vi "Change Label Popup.vi"(8 "error in":errorcluster, 11 "Label In":string) -> (0 "error out":errorcluster, 3 "Label Out":string)   [LabVIEW 2019]
doc: "All Rights Reserved © 2017 SyncSols"
uses:
  <vilib>/Utility/inputDevices.llb/keyboardAcquire.vi
panel:
  in  "Label Name":string
  # "<<Enter to Save the Changes>>"
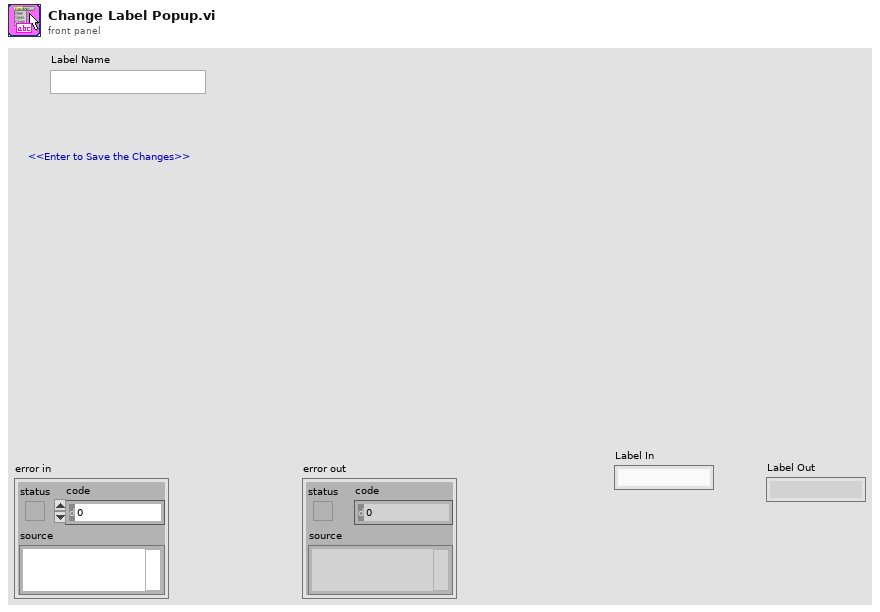
[diagram p1: front panel]
types:
  T1 = enum16{"0", "1", "2", "3", "4", "5", "6", "7", "8", "9", "A", "B", "C", "D", "E", "F", "G", "H", "I", "J", "K", "L", "M", "N", "O", "P", "Q", "R", "S", "T", "U", "V", "W", "X", "Y", "Z", "F1", "F2", "F3", "F4", "F5", "F6", "F7", "F8", "F9", "F10", "F11", "F12", "F13", "F14", "F15", "ADD", "BACK", "BACKSLASH", "CAPITAL", "COMMA", "DECIMAL", "DELETE", "DIVIDE", "DOWN", "END", "EQUALS", "ESCAPE", "GRAVE (`)", "HOME", "INSERT", "LBRACKET", "LCONTROL", "LEFT", "L ALT", "LSHIFT", "LWIN", "MINUS", "MULTIPLY", "NEXT", "NUMLOCK", "NUMPAD_0", "NUMPAD_1", "NUMPAD_2", "NUMPAD_3", "NUMPAD_4", "NUMPAD_5", "NUMPAD_6", "NUMPAD_7", "NUMPAD_8", "NUMPAD_9", "PAUSE", "PERIOD", "PRIOR (PG UP)", "RBRACKET", "RCONTROL", "RETURN", "RIGHT", "R ALT", "RSHIFT", "RWIN", "SCROLL", "SEMICOLON", "SLASH", "SPACE", "SUBTRACT", "TAB", "UP", "ENTER (num pad)", "' (quote)"}
  T2 = enum16{"0", "1", "2", "3", "4", "5", "6", "7", "8", "9", "A", "B", "C", "D", "E", "F", "G", "H", "I", "J", "K", "L", "M", "N", "O", "P", "Q", "R", "S", "T", "U", "V", "W", "X", "Y", "Z", "F1", "F2", "F3", "F4", "F5", "F6", "F7", "F8", "F9", "F10", "F11", "F12", "F13", "F14", "F15", "ADD", "BACK", "BACKSLASH", "CAPITAL", "COMMA", "DECIMAL", "DELETE", "DIVIDE", "DOWN", "END", "EQUALS", "ESCAPE", "GRAVE (`)", "HOME", "INSERT", "LBRACKET", "LCONTROL", "LEFT", "L ALT", "LSHIFT", "LWIN", "MINUS", "MULTIPLY", "NEXT", "NUMLOCK", "NUMPAD_0", "NUMPAD_1", "NUMPAD_2", "NUMPAD_3", "NUMPAD_4", "NUMPAD_5", "NUMPAD_6", "NUMPAD_7", "NUMPAD_8", "NUMPAD_9", "PAUSE", "PERIOD", "PRIOR (PG UP)", "RBRACKET", "RCONTROL", "RETURN", "RIGHT", "R ALT", "RSHIFT", "RWIN", "SCROLL", "SEMICOLON", "SLASH", "SPACE", "SUBTRACT", "TAB", "UP", "ENTER (num pad)", "' (quote)"}[]
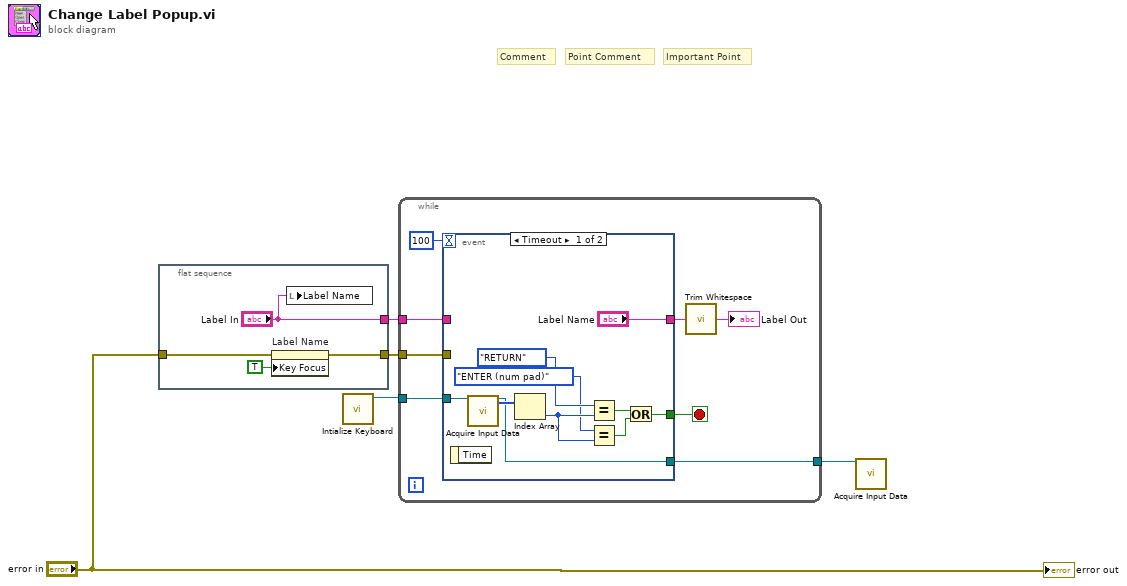
[diagram p0: block diagram]
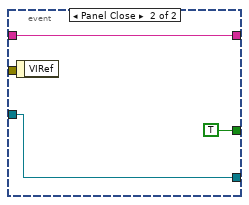
[diagram p2: hidden frame]
diagram:
  # "Important Point"
  # "Point Comment"
  # "Comment"
  n1 = flat-sequence {
    tunnel: "error in" -> [w8]
    tunnel: ["Label In"] -> w4
    tunnel: [w6] -> w1
    frame #0 {
      n2 = property on="Label Name" class="Str"(error in=w8, "Key Focus"=TRUE) -> (error out=w6:errorcluster)  [unwired: 1 in, 1 out]
      n3 = local write "Label Name"("Label In") -> ()
    }
  }
  n4 = call <vilib>:"Intialize Keyboard.vi"() -> ("device ID"=w3:refnum<k1>)  [unwired: 10 in, 1 out]
  n5 = while {
    tunnel: w4 -> [w14]
    tunnel: w3 -> [w13]
    tunnel: [w12] -> w2
    tunnel: w1 -> [w11]
    stop <- w15 stop-if-true
    n6 = event shown="[0] Timeout" {
      selector: _ -> [_ _]
      dyn-events: _ -> [_ _]
      timeout: 100 -> [_ _]
      tunnel: ["Label Name" w29] -> w17
      tunnel: [w21 TRUE] -> w15
      tunnel: w14 -> [_ w29]
      tunnel: w13 -> [w26 w28]
      tunnel: [w18 w28] -> w12
      tunnel: w11 -> [_ _]
      event Timeout {
        n7 = event-data() -> ()  [unwired: 1 in, 1 out]
        n8 = call-poly <vilib>:"Acquire Input Data.vi"("device ID"=w26) -> ("device ID"=w18:refnum<k1>, "keys pressed"=w25:T2)  [unwired: 16 in, 1 out]
        n9 = Index Array(array=w25) -> (element=w23:T1)  [unwired: 1 in]
        n10 = Equal?(x=T1."RETURN" ("keyType 3"), y=w23) -> (x = y?=w20:bool)
        n11 = Equal?(x=T1."ENTER (num pad)" ("keyType 3"), y=w23) -> (x = y?=w19:bool)
        n12 = Or(x=w20, y=w19) -> (x .or. y?=w21:bool)
      }
      event Panel Close {
        n13 = event-data() -> ()  [unwired: 1 in, 1 out]
      }
    }
    n14 = call <vilib>:"Trim Whitespace.vi"("string"=w17) -> ("trimmed string"=→"Label Out":string)  [unwired: 1 in]
  }
  n15 = call-poly <vilib>:"Acquire Input Data.vi"("device ID"=w2) -> ()  [unwired: 16 in, 3 out]
  "error out" <- "error in"
